vi "DB UI - Logon (Popup).vi"(9 "User":string, 10 "Application":string="SRTRS", 11 "Main.vi VI's Path":path=path "C:/Users/CK/workspace/LabVIEW/Stress Relief Temperature Recording") -> ()   [LabVIEW 2013]
uses:
  <vilib>/Utility/miscctls.llb/LVPointTypeDef.ctl
panel:
  out "Ref Error":errorcluster
  out "error out":errorcluster
  out "Logon Loop":i32
  out "Front Panel Window:State":T1(ring)
  out "Execution:State":T2(ring)
  # "C:\\Users\\CK\\workspace\\LabVIEW\\Stress Relief Temperature Recording\\VIs\\Main.vi"
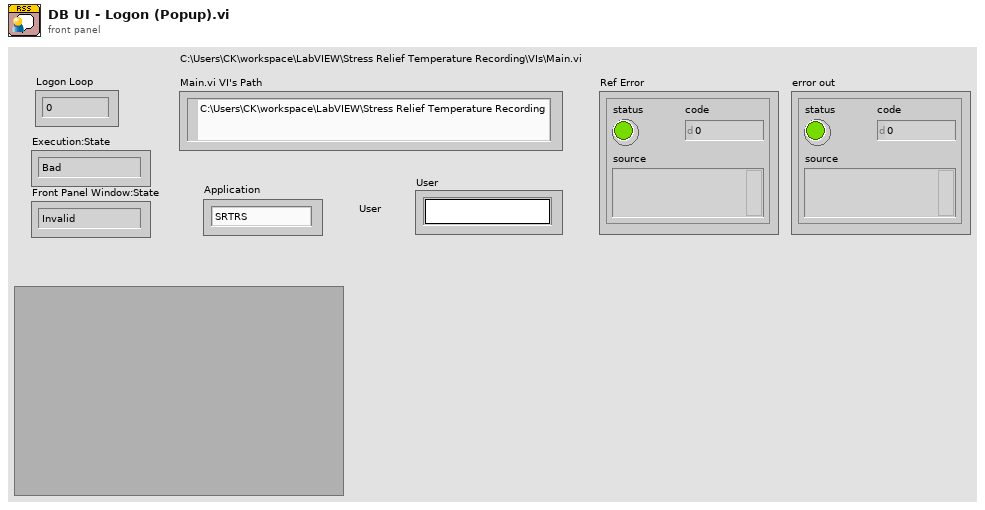
[diagram p1: front panel]
types:
  T1 = enum32{"Invalid", "Standard", "Closed", "Hidden", "Minimized", "Maximized"}
  T2 = enum32{"Bad", "Idle", "Run top level", "Running"}
  T3 = enum16{"Always On", "Always Off", "Off While Running"}
  T4 = typedef "LVPointTypeDef.ctl" = cluster{"Horizontal":i16, "Vertical":i16}
  T5 = enum8{"Enabled", "Disabled", "Disabled and Grayed Out"}
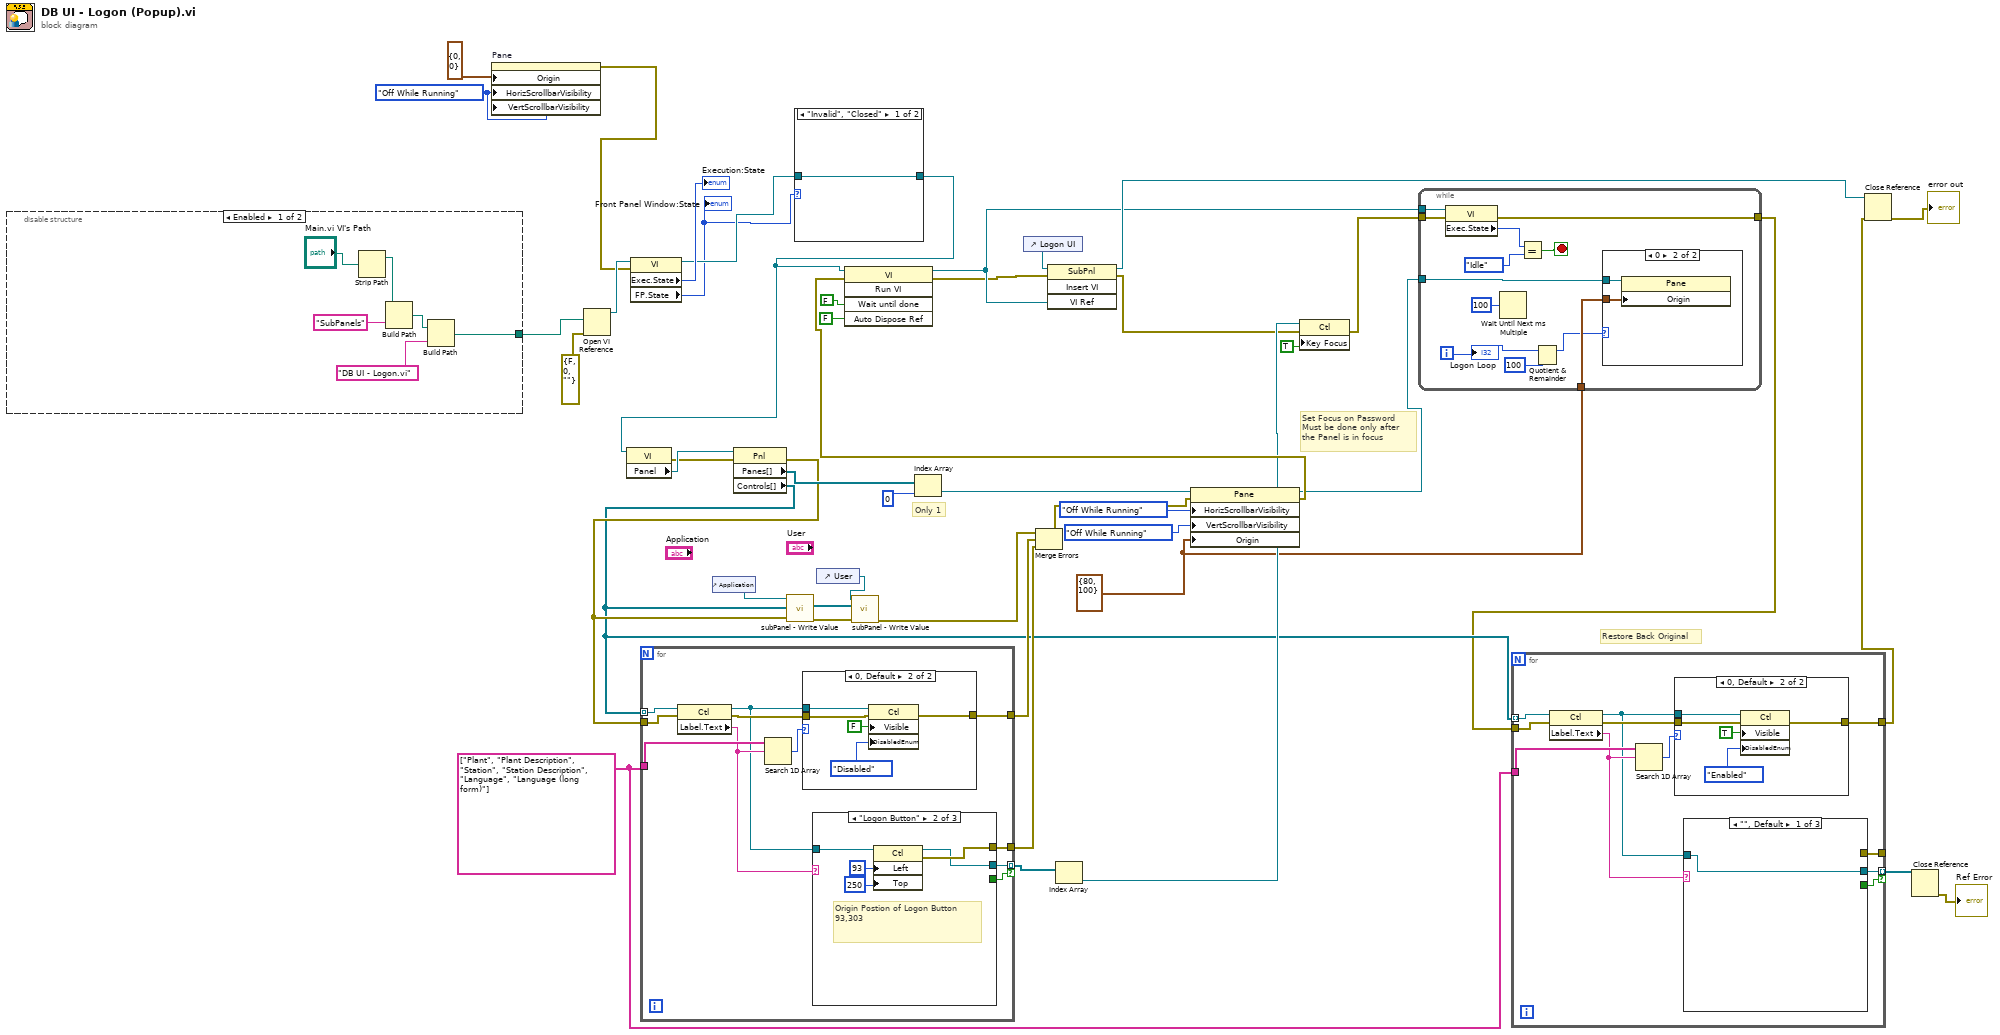
[diagram p0: block diagram]
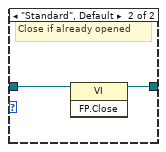
[diagram p2: hidden frame]
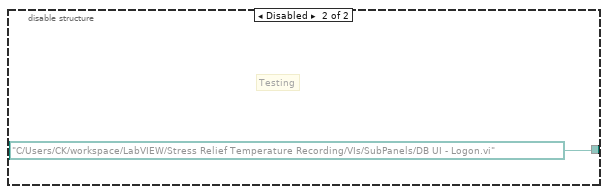
[diagram p3: hidden frame]
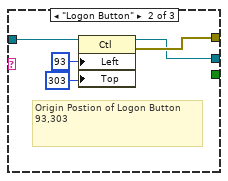
[diagram p4: hidden frame]
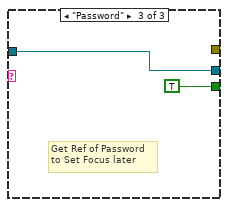
[diagram p5: hidden frame]
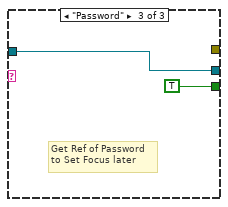
[diagram p8: hidden frame]
diagram:
  w13 = string[] ["Plant", "Plant Description", "Station", "Station Description", "Language", "Language (long form)"]
  w32 = T3."Off While Running" ("Horizontal Scrollbar Visibility")
  w2 = T4 {"Horizontal"=80, "Vertical"=100} ("Origin")
  # "Only 1"
  # "Restore Back Original"
  # "Set Focus on Password\nMust be done only after \nthe Panel is in focus"
  n1 = disable-structure shown="Enabled" {
    disable-tunnel: [w51 path "C:/Users/CK/workspace/LabVIEW/Stress Relief Temperature Recording/VIs/SubPanels/DB UI - Logon.vi" ("path")] -> w46
    frame Enabled {
      n2 = Strip Path(path="Main.vi VI's Path") -> (stripped path=w48:path)  [unwired: 1 out]
      n3 = Build Path(base path=w48, name or relative path="SubPanels") -> (appended path=w52:path)
      n4 = Build Path(base path=w52, name or relative path="DB UI - Logon.vi") -> (appended path=w51:path)
    }
    frame Disabled {
      # "Testing"
    }
  }
  n5 = property on="Pane" class="Pane"("Origin"=T4 {"Horizontal"=0, "Vertical"=0}, "HorizScrollbarVisibility"=w32, "VertScrollbarVisibility"=w32) -> (error out=w10:errorcluster)  [unwired: 2 in, 1 out]
  n6 = Open VI Reference(vi path=w46, error in (no error)=errorcluster {"status"=FALSE, "code"=0, "source"=""} ("error constant")) -> (vi reference=w45:refnum<vi>)  [unwired: 4 in, 1 out]
  n7 = property class="VI"(reference=w45, error in=w10) -> (reference out=w8:refnum<vi>, "Exec.State"=→"Execution:State":T2, "FP.State"=w6:T1)  [unwired: 1 out]
  "Front Panel Window:State" <- w6
  n8 = control-ref of="Application"() -> (w21:refnum<vi>)
  n9 = case shown="\"Invalid\", \"Closed\"" w6 {
    tunnel: w8 -> [w55 w57]
    tunnel: [w55 w56] -> w7
    frame "Invalid", "Closed" {
    }
    frame "Standard", Default {
      # "Close if already opened"
      n10 = invoke class="VI" method="FP.Close"(reference=w57) -> (reference out=w56:refnum<vi>)  [unwired: 2 in, 2 out]
    }
  }
  n11 = property class="VI"(reference=w7) -> (error out=w39:errorcluster, "Panel"=w40:refnum<vi>)  [unwired: 1 in, 1 out]
  n12 = property class="Pnl"(reference=w40, error in=w39) -> (error out=w28:errorcluster, "Panes[]"=w38:refnum<vi>[], "Controls[]"=w15:refnum<vi>[])  [unwired: 1 out]
  n13 = for {
    tunnel: w15 -> [w68] mode=indexing
    tunnel: [w67] -> w30
    tunnel: w28 -> [w65]
    tunnel: w13 -> [w64]
    tunnel: [w60] -> w26
    tunnel: [w59] -> w18 mode=indexing if=w58
    n14 = property class="Ctl"(reference=w68, error in=w65) -> (reference out=w61:refnum<vi>, error out=w66:errorcluster, "Label.Text"=w62:string)
    n15 = Search 1D Array(1D array=w64, element=w62) -> (index of element=w63:i32)  [unwired: 1 in]
    n16 = case shown="0, Default" w63 {
      tunnel: w61 -> [_ w82]
      tunnel: [w77 w80] -> w67
      tunnel: w66 -> [w77 w79]
      frame -1 {
      }
      frame 0, Default {
        n17 = property class="Ctl"(reference=w82, error in=w79, "Visible"=FALSE, "DisabledEnum"=T5."Disabled" ("Disabled")) -> (error out=w80:errorcluster)  [unwired: 1 out]
      }
    }
    n18 = case shown="\"Logon Button\"" w62 {
      tunnel: w61 -> [w69 w74 w75]
      tunnel: [_ w73 _] -> w60
      tunnel: [w69 w70 w75] -> w59
      tunnel: [_ _ TRUE] -> w58
      frame "", Default {
      }
      frame "Logon Button" {
        # "Origin Postion of Logon Button\n93,303"
        n19 = property class="Ctl"(reference=w74, "Left"=93 ("Position:Left"), "Top"=250 ("Position:Top")) -> (reference out=w70:refnum<vi>, error out=w73:errorcluster)  [unwired: 1 in]
      }
      frame "Password" {
        # "Get Ref of Password\nto Set Focus later"
      }
    }
  }
  n20 = call "subPanel - Write Value.vi"("Error In"=w28, "CtlRef Controls[]"=w15, "Pnl Control"=w21) -> ("Error Out"=w25:errorcluster, "CtlRef Controls[]"=w23:refnum<vi>[])  [unwired: 6 in, 1 out]
  n21 = control-ref of="User"() -> (w22:refnum<vi>)
  n22 = call "subPanel - Write Value.vi"("Error In"=w25, "CtlRef Controls[]"=w23, "Pnl Control"=w22) -> ("Error Out"=w24:errorcluster)  [unwired: 6 in, 2 out]
  n23 = Index Array(array=w38, index=0) -> (element=w35:refnum<vi>)
  n24 = control-ref of="Logon UI"() -> (w34:refnum<vi>)
  n25 = Merge Errors(w24, w30, w26) -> (w29:errorcluster)
  n26 = Index Array(array=w18) -> (element=w17:refnum<vi>)  [unwired: 1 in]
  n27 = property class="Pane"(reference=w35, error in=w29, "HorizScrollbarVisibility"=T3."Off While Running" ("Horizontal Scrollbar Visibility"), "VertScrollbarVisibility"=T3."Off While Running" ("Horizontal Scrollbar Visibility"), "Origin"=w2) -> (reference out=w3:refnum<vi>, error out=w31:errorcluster)
  n28 = invoke class="VI" method="Run VI"(reference=w7, error in=w31, "Wait until done"=FALSE ("Wait Until Done"), "Auto Dispose Ref"=FALSE ("Auto Dispose Reference")) -> (reference out=w41:refnum<vi>, error out=w20:errorcluster)  [unwired: 1 in, 3 out]
  n29 = invoke on="Invoke Node" class="SubPnl" method="Insert VI"(reference=w34, error in=w20, "VI Ref"=w41) -> (reference out=w42:refnum<vi>, error out=w16:errorcluster)  [unwired: 1 in, 2 out]
  n30 = property class="Ctl"(reference=w17, error in=w16, "Key Focus"=TRUE) -> (error out=w11:errorcluster)  [unwired: 1 out]
  n31 = while {
    tunnel: w41 -> [w94]
    tunnel: w11 -> [w93]
    tunnel: [w89] -> w14
    tunnel: w3 -> [w88]
    tunnel: w2 -> [w84]
    i -> [w86]
    stop <- w87 stop-if-true
    n32 = property class="VI"(reference=w94, error in=w93) -> (error out=w89:errorcluster, "Exec.State"=w92:T2)  [unwired: 1 out]
    n33 = Wait Until Next ms Multiple(millisecond multiple=u32 100) -> ()  [unwired: 1 out]
    n34 = Equal?(x=w92, y=T2."Idle" ("Execution:State")) -> (x = y?=w87:bool)
    n35 = Quotient & Remainder(x=w86, y=100) -> (x-y*floor(x/y)=w83:i32)  [unwired: 1 out]
    n36 = case shown="0" w83 {
      tunnel: w88 -> [_ w96]
      tunnel: w84 -> [_ w95]
      frame 1, Default {
      }
      frame 0 {
        n37 = property class="Pane"(reference=w96, "Origin"=w95) -> ()  [unwired: 1 in, 2 out]
      }
    }
    "Logon Loop" <- w86
  }
  n38 = for {
    tunnel: w15 -> [w107] mode=indexing
    tunnel: [w106] -> w12
    tunnel: w14 -> [w104]
    tunnel: w13 -> [w103]
    tunnel: [w99] -> _
    tunnel: [w98] -> w5 mode=indexing if=w97
    n39 = property class="Ctl"(reference=w107, error in=w104) -> (reference out=w100:refnum<vi>, error out=w105:errorcluster, "Label.Text"=w101:string)
    n40 = Search 1D Array(1D array=w103, element=w101) -> (index of element=w102:i32)  [unwired: 1 in]
    n41 = case shown="0, Default" w102 {
      tunnel: w100 -> [_ w121]
      tunnel: [w116 w119] -> w106
      tunnel: w105 -> [w116 w118]
      frame -1 {
      }
      frame 0, Default {
        n42 = property class="Ctl"(reference=w121, error in=w118, "Visible"=TRUE, "DisabledEnum"=T5."Enabled" ("Disabled")) -> (error out=w119:errorcluster)  [unwired: 1 out]
      }
    }
    n43 = case shown="\"\", Default" w101 {
      tunnel: w100 -> [w108 w113 w114]
      tunnel: [_ w112 _] -> w99
      tunnel: [w108 w109 w114] -> w98
      tunnel: [_ _ TRUE] -> w97
      frame "", Default {
      }
      frame "Logon Button" {
        # "Origin Postion of Logon Button\n93,303"
        n44 = property class="Ctl"(reference=w113, "Left"=93 ("Position:Left"), "Top"=303 ("Position:Top")) -> (reference out=w109:refnum<vi>, error out=w112:errorcluster)  [unwired: 1 in]
      }
      frame "Password" {
        # "Get Ref of Password\nto Set Focus later"
      }
    }
  }
  n45 = Close Reference(reference=w42, error in (no error)=w12) -> (error out=→"error out":errorcluster)
  n46 = Close Reference(reference=w5) -> (error out=→"Ref Error":errorcluster)  [unwired: 1 in]
